vi "getRFOutputvi.vi"(8 "error in (no error)":errorcluster, 11 "RfOutputData in":refnum<class "RfOutputData.lvclass">) -> (0 "error out":errorcluster, 2 "DDSOutput":refnum<class "DDSOutput.lvclass">, 3 "RfOutputData out":refnum<class "RfOutputData.lvclass">)   [LabVIEW 2011, in "DataMappers.lvlib" / "RfOutputData.lvclass"]
uses:
  RfOutputData.lvclass
  Hal/Channels/DDSOutput/Generic/DDSOutput.lvclass
  RfOutputData.lvclass/RfOutputData.ctl
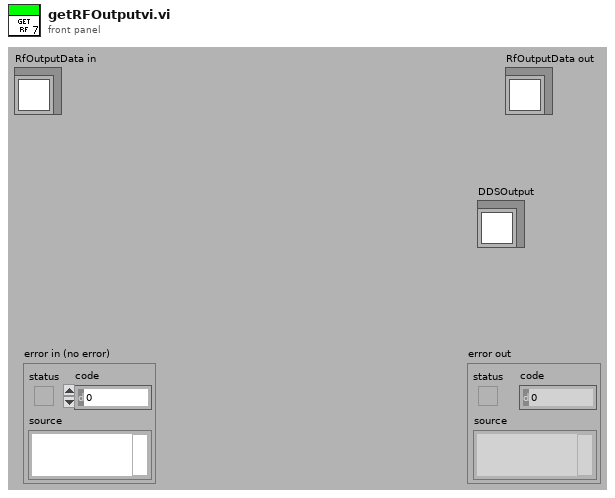
[diagram p1: front panel]
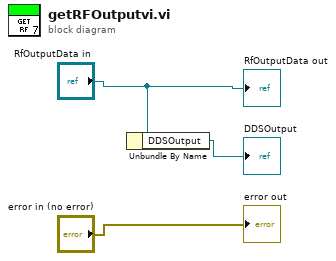
[diagram p0: block diagram]
diagram:
  n1 = Unbundle By Name("RfOutputData in") -> ("DDSOutput"=→"DDSOutput":refnum<class "DDSOutput.lvclass">)
  "error out" <- "error in (no error)"
  "RfOutputData out" <- "RfOutputData in"
